vi "Get Library Names.vi"(8 "error in (no error)":errorcluster, 9 "Override Name":string, 10 "Version":T1, 11 "Project Path":path) -> (0 "error out":errorcluster, 1 "Versioned Library (no extension)":string, 2 "Versioned Library":string, 3 "Library":string)   [LabVIEW 2021, in "CIF Build Actions.lvlib"]
uses:
  CIF Build Actions.lvlib
  CIFCore/Common/Typedef/Errors.ctl
  <vilib>/CIF Foundation/CIF Utilities/Errors/Append Error Location.vi
  CIFCore/Common/CIFCoreCommon.lvlib
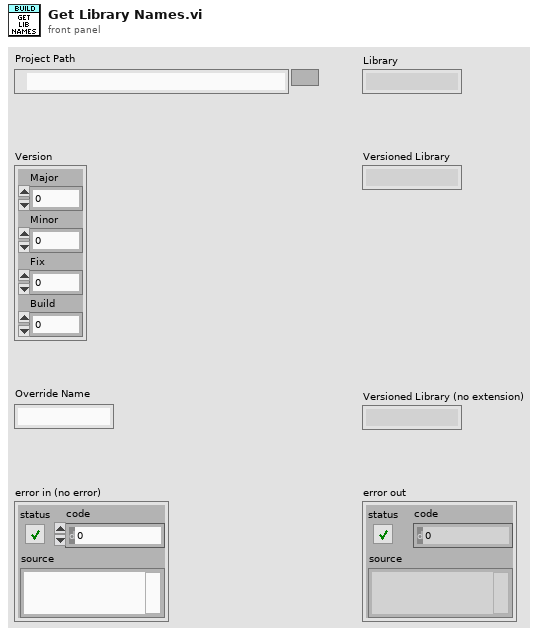
[diagram p1: front panel]
types:
  T1 = cluster{"Major":u16, "Minor":u16, "Fix":u16, "Build":u16}
  T2 = typedef "CIFCoreCommon.lvlib/Errors.ctl" = enum16{"Invalid Clock ID", "Long Sleep", "gRPC Server Not Found", "Config Parse", "Timestamp Wrap", "Delayed Execution", "Duplicate Channel", "Missing Channel", "Incorrect Type", "Flatten Error", "Unflatten Data", "Unique Name", "Plugin Not Found", "Plugin Type Not Found", "Plugin Version Not Found", "Manager Not Found", "Numerical Issue", "Time Jump", "Clock ID Match", "Channel Length", "Plugin Connection", "gRPC Server Connection", "PPL Name Match", "Build", "Config Log Parse", "Plugin Load", "UI Subpanel Load", "Python Name", "Invalid Name"}
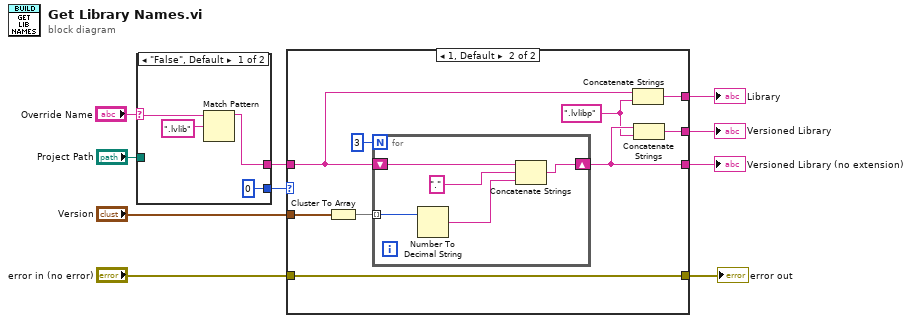
[diagram p0: block diagram]
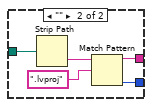
[diagram p2: hidden frame]
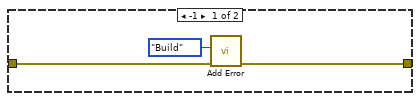
[diagram p3: hidden frame]
diagram:
  n1 = case shown="\"False\", Default" "Override Name" {
    selector: "Override Name" -> [w13 _]
    tunnel: "Project Path" -> [_ w17]
    tunnel: [w11 w16] -> w5
    tunnel: [0 ("offset past match") w15] -> w4
    frame "False", Default {
      n2 = Match Pattern(string=w13, regular expression=".lvlib") -> (before substring=w11:string)  [unwired: 1 in, 3 out]
    }
    frame "" {
      n3 = Strip Path(path=w17) -> (name=w18:string)  [unwired: 1 out]
      n4 = Match Pattern(string=w18, regular expression=".lvproj") -> (before substring=w16:string, offset past match=w15:i32)  [unwired: 1 in, 2 out]
    }
  }
  n5 = case shown="1, Default" w4 {
    tunnel: "Version" -> [_ w31]
    tunnel: [_ w28] -> w9
    tunnel: [_ w27] -> w8
    tunnel: [_ w26] -> w6
    tunnel: w5 -> [_ w25]
    tunnel: "error in (no error)" -> [w22 w23]
    tunnel: [w21 w23] -> w2
    frame -1 {
      n6 = call "Add Error.vi"("error in (no error)"=w22, "Error"=Errors."Build") -> ("error out"=w21:errorcluster)  [unwired: 9 in]
    }
    frame 1, Default {
      w24 = ".lvlibp" ("regular expression")
      n7 = Cluster To Array(cluster=w31) -> (array=w29:u16[])
      n8 = for {
        N: 3 -> [_]
        tunnel: w29 -> [w36] mode=indexing
        shift-right: [w32] -> w28
        shift-left: w25 -> [w35]
        n9 = Number To Decimal String(number=w36) -> (decimal integer string=w34:string)  [unwired: 1 in]
        n10 = Concatenate Strings(w35, "." ("string"), w34) -> (w32:string)
      }
      n11 = Concatenate Strings(w25, w24) -> (w26:string)
      n12 = Concatenate Strings(w28, w24) -> (w27:string)
    }
  }
  "Versioned Library (no extension)" <- w9
  "Versioned Library" <- w8
  "Library" <- w6
  "error out" <- w2
